vi "PR Set Time Out.vi"(0 "Seconds":i32) -> ()   [LabVIEW 2022 SP3, in "BS6006PRPLUS.lvlib"]
doc: "The function sets the timeout for acquiring signals.\n\n\nextern \"C\" BS6006PRPLUS_API void __cdecl PR_SetTimeOut(int Seconds);"
uses:
  BS6006PRPLUS.lvlib
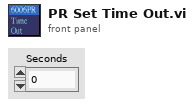
[diagram p1: front panel]
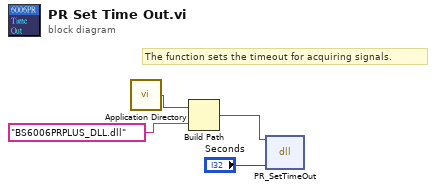
[diagram p0: block diagram]
diagram:
  # "The function sets the timeout for acquiring signals."
  n1 = call <vilib>:"Application Directory.vi"() -> ("Application Directory"=w3:path)
  n2 = Build Path(base path=w3, name or relative path="BS6006PRPLUS_DLL.dll") -> (appended path=w1:path)
  n3 = dll-call lib="E:/Broadsound_Program/PulserReceiver/6006PR PLUS/API/DLL/LabVIEW 15/VIs/BS6006PRPLUS_DLL.dlls" fn="PR_SetTimeOut"(path in=w1, "Seconds"="Seconds") -> ()  [unwired: 4 in, 2 out]
